vi "interfaz para quiz1.vi"() -> ()   [LabVIEW 2020]
panel:
  out "Respuesta":string
  in  "Array 2":string[](array[string])=["hola", "papa", "aloha"]
  in  "Ingreso de comandos":string
  in  "ENVIAR":bool
  out "Comando evaluado":string
  out "Arreglo a evaluar":string
  # "INTERFAZ"
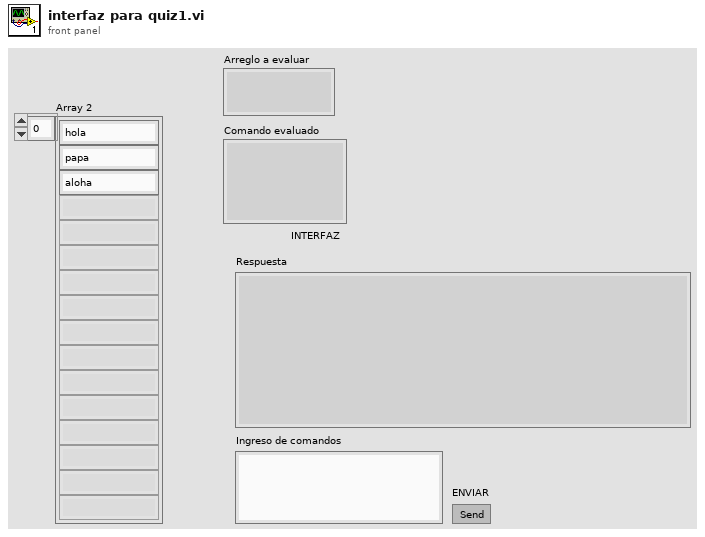
[diagram p1: front panel]
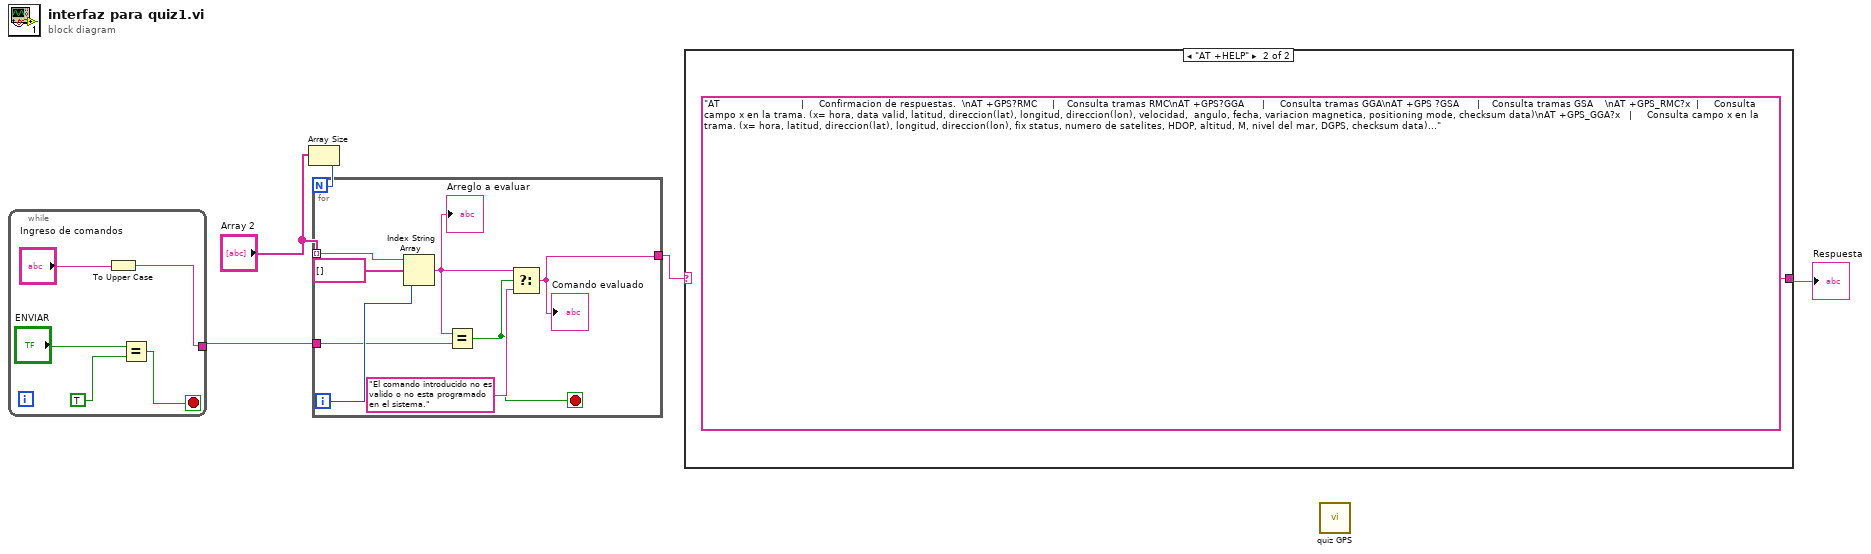
[diagram p0: block diagram]
diagram:
  n1 = while {
    tunnel: [w6] -> w4
    stop <- w8 stop-if-true
    n2 = To Upper Case(1:"Ingreso de comandos") -> (0:w6:string)
    n3 = Equal?(x="ENVIAR", y=TRUE) -> (x = y?=w8:bool)
  }
  n4 = Array Size(array="Array 2") -> (size(s)=w5:i32)
  n5 = for {
    N: w5 -> [_]
    tunnel: "Array 2" -> [w17] mode=indexing
    tunnel: w4 -> [w13]
    tunnel: [w11] -> w2
    i -> [w18]
    stop <- w12 stop-if-true
    n6 = Index String Array(1:w18, 2:string[] [] ("string array"), 3:w17) -> (0:w15:string)
    "Arreglo a evaluar" <- w15
    n7 = Equal?(x=w15, y=w13) -> (x = y?=w12:bool)
    n8 = Select(t=w15, s=w12, f="El comando introducido no es valido o no esta programado en el sistema.") -> (s? t:f=w11:string)
    "Comando evaluado" <- w11
  }
  n9 = case shown="\"AT +HELP\"" w2 {
    tunnel: [_ "AT                           |     Confirmacion de respuestas.  \nAT +GPS?RMC     |    Consulta tramas RMC\nAT +GPS?GGA      |     Consulta tramas GGA\nAT +GPS ?GSA      |    Consulta tramas GSA    \nAT +GPS_RMC?x  |     Consulta campo x en la trama. (x= hora, data valid, latitud, direccion(lat), longitud, direccion(lon), velocidad,  angulo, fecha, variacion magnetica, positioning mode, checksum data)\nAT +GPS_GGA?x   |     Consulta campo x en la trama. (x= hora, latitud, direccion(lat), longitud, direccion(lon), fix status, numero de satelites, HDOP, altitud, M, nivel del mar, DGPS, checksum data)\nAT +GPS_GSA?x    |     Consulta campo x en la trama. (x= mode, fixstatus, su1, su2, su3, su4, su5, su6, su7, su8 ,su9, su10, su11, su12, PDOP, HDOP, VDOP, checksumdata )  \nAT +TIMEPC          |     Consulta la hora actual de tu pc.\nAT +CAMBIARTIEMPO |  Cambia cada cuanto tiempo aumenta la variable contador.\nAT +LEECONTADOR | Lee la variable contador.\nAT +LEERLEDS        |  Lee estado de los led. \nAT+MODIFLEDS      | Modifica el estado de los pulsadores de los leds.\n\n      \n           "] -> w1
    frame "False", Default {
    }
    frame "AT +HELP" {
    }
  }
  "Respuesta" <- w1
  n10 = call "quiz GPS.vi"() -> ()  [unwired: 1 in, 3 out]
